vi "1.vi"() -> ()   [LabVIEW 2017]
panel:
  out "数值":dbl
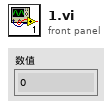
[diagram p1: front panel]
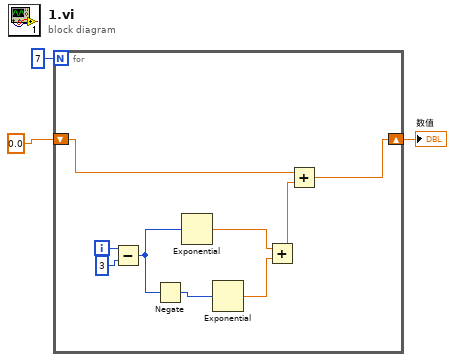
[diagram p0: block diagram]
diagram:
  n1 = for {
    N: 7 -> [_]
    shift-right: [w4] -> w1
    shift-left: 0.0 -> [w6]
    i -> [w12]
    n2 = Subtract(x=w12, y=3) -> (x-y=w10:i32)
    n3 = Negate(x=w10) -> (-x=w9:i32)
    n4 = Exponential(1:w10) -> (0:w7:dbl)
    n5 = Exponential(1:w9) -> (0:w8:dbl)
    n6 = Add(x=w7, y=w8) -> (x+y=w5:dbl)
    n7 = Add(x=w6, y=w5) -> (x+y=w4:dbl)
  }
  "数值" <- w1
